vi "UMLEditor_PlugInRefVI.vi"(8 "error in (no error)":errorcluster) -> (0 "error out":errorcluster, 1 "reference":refnum<class "Graph.lvclass">, 2 "cancelled":bool, 3 "diagramType":T1)   [LabVIEW 2016]
uses:
  <resource>/Framework/Providers/Open_GDS/UML/Graph_class/private/diagramType.ctl
  <resource>/Framework/Providers/Open_GDS/UML/Graph_class/Graph.lvclass
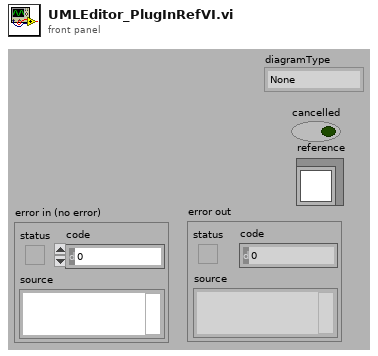
[diagram p1: front panel]
types:
  T1 = typedef "Graph.lvclass/diagramType.ctl" = enum16{"None", "Class", "Sequency", "State", "UseCase", "DQMH-Module"}
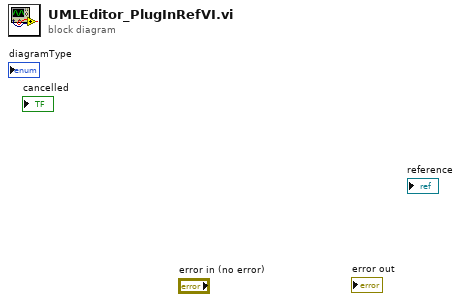
[diagram p0: block diagram]
diagram:
